vi "Read Time First Active.vi"(8 "error in (no error)":errorcluster, 11 "Button in":refnum<class "Button.lvclass">) -> (0 "error out":errorcluster, 2 "Time First Active":timestamp, 3 "Button out":refnum<class "Button.lvclass">)   [LabVIEW 2019, in "Button.lvclass"]
uses:
  Button.lvclass
  Button.lvclass/Button.ctl
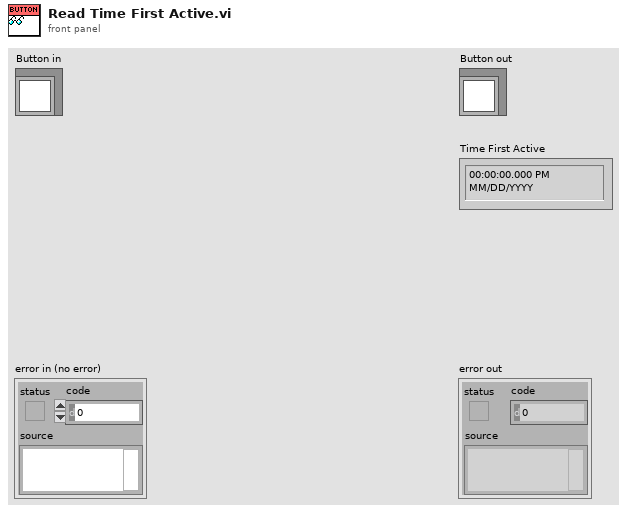
[diagram p1: front panel]
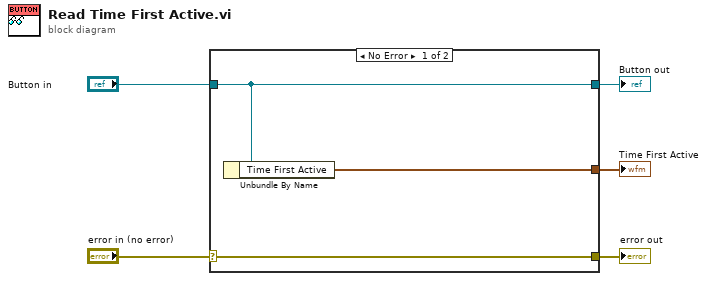
[diagram p0: block diagram]
diagram:
  n1 = case shown="No Error" "error in (no error)" {
    selector: "error in (no error)" -> [w8 w9]
    tunnel: [w8 w9] -> w4
    tunnel: [w7 w10] -> w2
    tunnel: "Button in" -> [w7 w10]
    tunnel: [w6 _] -> w1
    frame No Error {
      n2 = Unbundle By Name(w7) -> ("Time First Active"=w6:timestamp)
    }
    frame Error {
    }
  }
  "error out" <- w4
  "Button out" <- w2
  "Time First Active" <- w1
